vi "XIPIN_ZYNQ7_Processing_System_BFM_2_0.vi"   [LabVIEW 2017]
doc: "ZYNQ7 Processing System BFM\n------------------------------------\n<b>Need License</b> : No\n<b>Interface</b> : AXI4"
uses:
  <vilib>/rvi/XilinxIP/XIPIN_XNode/niFpgaXIPIN.xnode
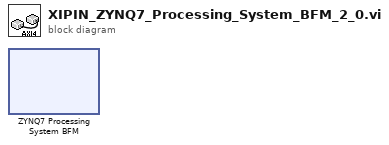
[diagram p0: block diagram]
diagram:
  n1 = xnode ("ZYNQ7 Processing System BFM")() -> ()
